vi "Configure Dialog.vi"(7 "Data in":path, 11 "Path Selector in":refnum<class "MGI Path Selector.lvclass">) -> (2 "Changed?":bool, 3 "Path Selector out":refnum<class "MGI Path Selector.lvclass">, 5 "Data out":path)   [LabVIEW 2020, in "MGI Path Selector.lvclass"]
uses:
  <userlib>/_MGI/User Interface/Path Selector XControl/Class Hierarchy/MGI Path Selector.lvclass
  <userlib>/_MGI/User Interface/Path Selector XControl/Control Style Enum.ctl
  <userlib>/_MGI/User Interface/Path Selector XControl/Class Hierarchy/MGI Path Selector.lvclass/MGI Path Selector.ctl
  <userlib>/_MGI/User Interface/Path Selector XControl/MGI Path Selector.xctl
panel:
  in  "Control Style":T1 caption="Control Style of File Selector"
  in  "Done":bool
  # "This dialog allows configuration of the File Selector.  This dialog should be overridden by the child class.\nThe file selector is a combo box that shows files from a directory and allows the user to select a file.    The directory containing the files (file directory) is typically the folder containing the file last selected by the user.  The File Selector remembers which file is selected by the user by saving this information to a file."
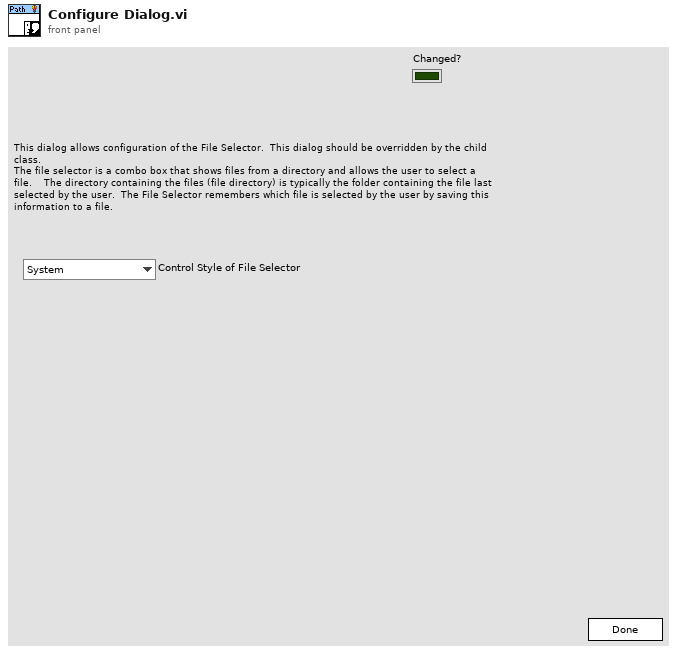
[diagram p1: front panel]
types:
  T1 = typedef "MGI Path Selector.xctl/Control Style Enum.ctl" = enum16{"System", "Modern", "Classic", "Silver"}
  T2 = enum16{"Left Button", "Center Button", "Right Button", "Window Close"}
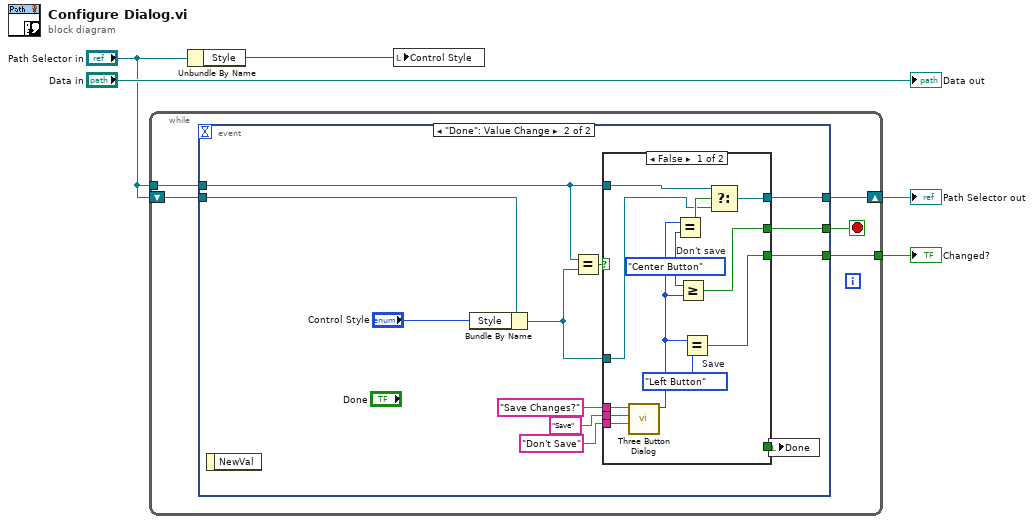
[diagram p0: block diagram]
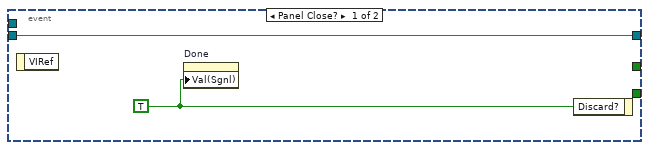
[diagram p2: hidden frame]
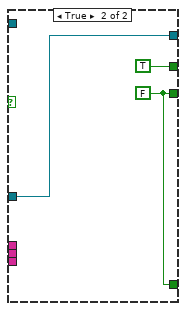
[diagram p3: hidden frame]
diagram:
  n1 = while {
    shift-right: [w6] -> w4
    shift-left: "Path Selector in" -> [w10]
    tunnel: "Path Selector in" -> [w9]
    tunnel: [w7] -> w2
    stop <- w8 stop-if-true
    n2 = event shown="[1] \"Done\": Value Change" {
      selector: _ -> [_ _]
      dyn-events: _ -> [_ _]
      timeout: _ -> [_ _]
      tunnel: w10 -> [w12 w22]
      tunnel: w9 -> [_ w23]
      tunnel: [_ w17] -> w8
      tunnel: [_ w16] -> w7
      tunnel: [w12 w18] -> w6
      event Panel Close? {
        w11 = TRUE ("Discard?")
        n3 = event-data() -> ()  [unwired: 1 in, 1 out]
        n4 = property on="Done" class="Bool (strict)"("Val(Sgnl)"=w11) -> ()  [unwired: 2 in, 2 out]
        n5 = event-data("Discard?"=w11) -> ()  [unwired: 1 in, 1 out]
      }
      event "Done": Value Change {
        n6 = event-data() -> ()  [unwired: 1 in, 1 out]
        n7 = Bundle By Name(cluster=w22, "Style"="Control Style") -> (w14:refnum<class "MGI Path Selector.lvclass">)
        n8 = Equal?(x=w23, y=w14) -> (x = y?=w24:bool)
        n9 = case shown="False" w24 {
          tunnel: w23 -> [w30 _]
          tunnel: "Save Changes?" ("message") -> [w36 _]
          tunnel: "Save" ("Left Button Text (\"Yes\")") -> [w35 _]
          tunnel: "Don't Save" ("Center Button Text (\"No\")") -> [w34 _]
          tunnel: [w29 w37] -> w18
          tunnel: [w33 TRUE] -> w17
          tunnel: [w26 w38] -> w16
          tunnel: [_ w38] -> w15
          tunnel: w14 -> [w25 w37]
          frame False {
            w27 = T2."Left Button"  # Save
            w32 = T2."Center Button"  # Don't save
            n10 = call <vilib>:"Three Button Dialog.vi"("Center Button Text (\"No\")"=w34, "Left Button Text (\"Yes\")"=w35, "message"=w36) -> ("Which Button?"=w28:T2)  [unwired: 8 in]
            n11 = Equal?(x=w28, y=w32) -> (x = y?=w31:bool)
            n12 = Greater Or Equal?(x=w32, y=w28) -> (x >= y?=w33:bool)
            n13 = Equal?(x=w28, y=w27) -> (x = y?=w26:bool)
            n14 = Select(t=w30, s=w31, f=w25) -> (s? t:f=w29:refnum<class "MGI Path Selector.lvclass">)
          }
          frame True {
            w38 = FALSE
          }
        }
        n15 = local write "Done"(w15) -> ()
      }
    }
  }
  "Changed?" <- w2
  "Path Selector out" <- w4
  n16 = Unbundle By Name("Path Selector in") -> ("Style"=w1:T1)
  n17 = local write "Control Style"(w1) -> ()
  "Data out" <- "Data in"
